vi "Begin.vi"(8 "error in":errorcluster) -> (0 "error out":errorcluster)   [LabVIEW 2015]
doc: "Called before other user functions, this VI is expected to open initial I/O refnums, load in file data, and do all program initialization. Notice that the <B>error out</B> terminal is simply used for data flow. Wiring it to other structures or subVIs ensures that this VI runs first."
uses:
  <vilib>/Rock Robotics/SystemInterfaces/DIO/FPGA_DIOPWMChannel.ctl
  <vilib>/Rock Robotics/WPI/SafetyOutput/WPI_SafetyOutputConfigMenu.ctl
  <vilib>/Rock Robotics/WPI/DriverStation/WPI_DriverStationRobotMode2.ctl
  <vilib>/Rock Robotics/WPI/Joystick/WPI_JoystickDeviceEnum.ctl
  <vilib>/Rock Robotics/SystemInterfaces/DIO/FPGA_DIOChannel.ctl
  <vilib>/Rock Robotics/WPI/Encoder/WPI_EncoderType.ctl
  <vilib>/Rock Robotics/WPI/RobotDrive/WPI_RobotDriveOpen2MotorWithTalon.vi
  Robot Global Data.vi
  <vilib>/Rock Robotics/Network Tables/NT Write String Array.vi
  <vilib>/Rock Robotics/WPI/Counter/WPI_CounterDigitalInputToDigitalSource.vi
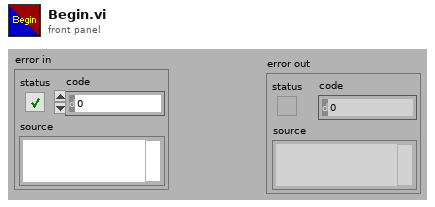
[diagram p1: front panel]
types:
  T1 = typedef "WPI_JoystickDeviceEnum.ctl" = enum16{"USB 0", "USB 1", "USB 2", "USB 3", "USB 4", "USB 5"}
  T2 = typedef "WPI_EncoderType.ctl" = enum16{"1x", "2x", "4x"}
  T3 = typedef "FPGA_DIOChannel.ctl" = enum8{"DIO 0", "DIO 1", "DIO 2", "DIO 3", "DIO 4", "DIO 5", "DIO 6", "DIO 7", "DIO 8", "DIO 9", "DIO MXP 0", "DIO MXP 1", "DIO MXP 2", "DIO MXP 3", "DIO MXP 4", "DIO MXP 5", "DIO MXP 6", "DIO MXP 7", "DIO MXP 8", "DIO MXP 9", "DIO MXP 10", "DIO MXP 11", "DIO MXP 12", "DIO MXP 13", "DIO MXP 14", "DIO MXP 15", "Invalid"}
  T4 = typedef "WPI_DriverStationRobotMode2.ctl" = enum16{"Autonomous Disabled", "Autonomous Enabled", "Teleop Disabled", "Teleop Enabled", "Disconnected", "Finish", "Test Disabled", "Test Enabled", "Emergency Stopped"}
  T5 = typedef "WPI_SafetyOutputConfigMenu.ctl" = enum16{"Enable", "Disable"}
  T6 = typedef "FPGA_DIOPWMChannel.ctl" = enum8{"PWM 0", "PWM 1", "PWM 2", "PWM 3", "PWM 4", "PWM 5", "PWM 6", "PWM 7", "PWM 8", "PWM 9", "PWM MXP 0", "PWM MXP 1", "PWM MXP 2", "PWM MXP 3", "PWM MXP 4", "PWM MXP 5", "PWM MXP 6", "PWM MXP 7", "PWM MXP 8", "PWM MXP 9", "Invalid"}
  T7 = typedef "WPI_JoystickDevRef.ctl" = cluster{"Device":T1}
  T8 = typedef "WPI_RobotDriveDevRef.ctl" = cluster{"DevStatus":errorcluster, "Motors[]":T9[], "Square Inputs":bool, "Max Output":dbl}
  T9 = typedef "WPI_MotorControlDeviceRef.ctl" = cluster{"DeviceStatus":errorcluster, "Type":T10, "PWM":cluster{"PWM Channel":T6, "DeadBand":T11}, "CAN":cluster{"Device Number":u8, "Control Mode":T12, "Semaphore":T13, "Max Vout":dbl, "TalonSRX Control Mode":T14}, "Invert":bool}
  T10 = typedef "WPI_MotorControlType.ctl" = enum16{"PWM", "CAN", "CANTalonSRX"}
  T11 = typedef "WPI_PWMDeadband.ctl" = cluster{"Name":string, "maxPositivePwm":i32, "minPositivePwm":i32, "centerPwm":i32, "maxNegativePwm":i32, "minNegativePwm":i32, "angularRange":u16}
  T12 = typedef "WPI_CANJaguar_ControlMode.ctl" = enum8{"Percent VBus", "Current", "Speed", "Position", "Voltage"}
  T13 = typedef "Semaphore RefNum" = refnum<k1>
  T14 = typedef "WPI_CANTalonSRX_APIControlMode.ctl" = enum8{"Percent VBus", "Speed", "Position", "Slave", "Unchanged / Invalid", "Voltage Compensation", "Current", "Motion Profile"}
  T15 = typedef "WPI_DigitalInputDevRef.ctl" = cluster{"DevStatus":errorcluster, "DIO Channel":T3}
  T16 = typedef "FPGA_CounterEncoderSourceConvertionLVSourceType.ctl" = cluster{"DevStatus":errorcluster, "AnalogTriggerMode?":bool, "DigitalMode":cluster{"DIO Channel":T17}, "AnalogTriggerMode":cluster{"AnalogTriggerIndex":T18, "OutputType":T19}}
  T17 = typedef "FPGA_DIODigitalSourceChannel.ctl" = enum8{"DIO 0", "DIO 1", "DIO 2", "DIO 3", "DIO 4", "DIO 5", "DIO 6", "DIO 7", "DIO 8", "DIO 9", "DIO MXP 0", "DIO MXP 1", "DIO MXP 2", "DIO MXP 3", "DIO MXP 4", "DIO MXP 5", "DIO MXP 6", "DIO MXP 7", "DIO MXP 8", "DIO MXP 9", "DIO MXP 10", "DIO MXP 11", "DIO MXP 12", "DIO MXP 13", "DIO MXP 14", "DIO MXP 15", "Disabled"}
  T18 = typedef "FPGA_AnalogTriggerIndex.ctl" = enum8{"Trig 0", "Trig 1", "Trig 2", "Trig 3", "Trig 4", "Trig 5", "Trig 6", "Trig 7", "Invalid"}
  T19 = typedef "FPGA_AnalogTriggerOutType.ctl" = enum16{"InWindow", "TriggerState", "Rising", "Falling"}
  T20 = typedef "WPI_EncoderDevRef.ctl" = cluster{"DevStatus":errorcluster, "EncoderIndex":T21, "CounterIndex":T22, "DistancePerCount":dbl, "Decoding Type":T2}
  T21 = typedef "FPGA_EncoderIdx.ctl" = enum8{"Enc 0", "Enc 1", "Enc 2", "Enc 3", "Enc 4", "Enc 5", "Enc 6", "Enc 7", "Invalid"}
  T22 = typedef "FPGA_CounterCtrSystemIndex.ctl" = enum8{"Ctr 0", "Ctr 1", "Ctr 2", "Ctr 3", "Ctr 4", "Ctr 5", "Ctr 6", "Ctr 7", "Invalid"}
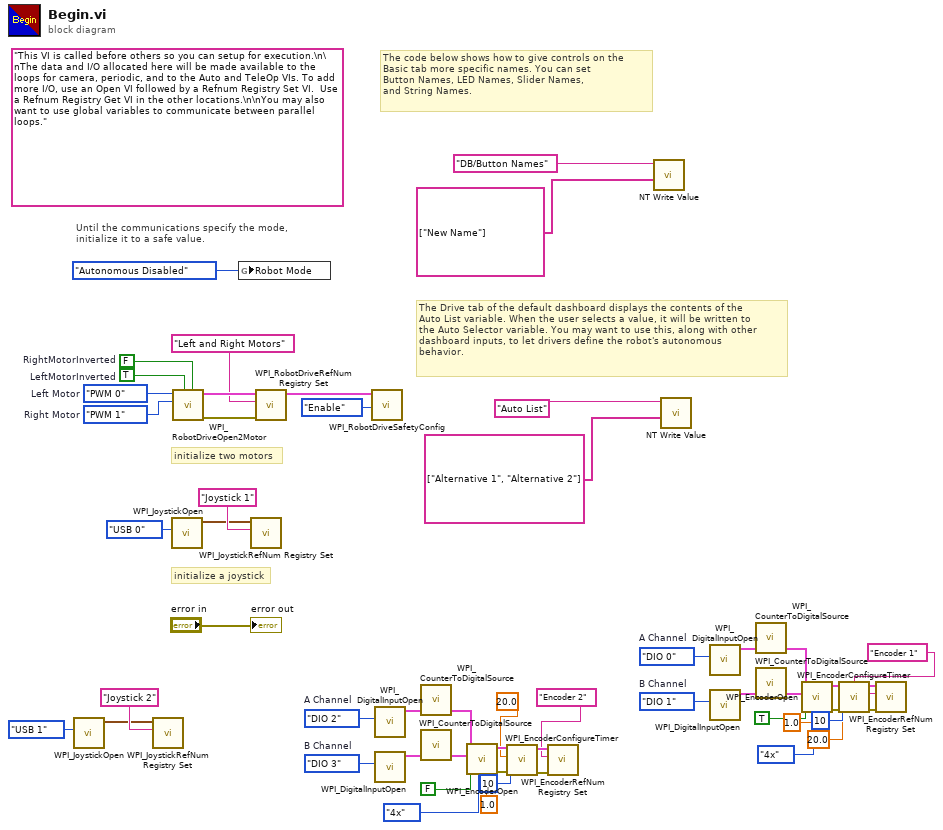
[diagram p0: block diagram]
diagram:
  w19 = FPGA_DIOChannel."DIO 3"  # B Channel
  w18 = FPGA_DIOChannel."DIO 2"  # A Channel
  w35 = FPGA_DIOChannel."DIO 1"  # B Channel
  w34 = FPGA_DIOChannel."DIO 0"  # A Channel
  (unwired) "This VI is called before others so you can setup for execution.\n\nThe data and I/O allocated here will be made available to the loops for camera, periodic, and to the Auto and TeleOp VIs. To add more I/O, use an Open VI followed by a Refnum Registry Set VI.  Use a Refnum Registry Get VI in the other locations.\n\nYou may also want to use global variables to communicate between parallel loops."
  w47 = FPGA_DIOPWMChannel."PWM 1"  # Right Motor
  w48 = FPGA_DIOPWMChannel."PWM 0"  # Left Motor
  w52 = TRUE  # LeftMotorInverted
  w53 = FALSE  # RightMotorInverted
  # "The Drive tab of the default dashboard displays the contents of the\nAuto List variable. When the user selects a value, it will be written to\nthe Auto Selector variable. You may want to use this, along with other\ndashboard inputs, to let drivers define the robot's autonomous\nbehavior."
  # "The code below shows how to give controls on the\nBasic tab more specific names. You can set\nButton Names, LED Names, Slider Names,\nand String Names."
  # "initialize a joystick"
  # "Until the communications specify the mode,\ninitialize it to a safe value."
  # "initialize two motors"
  n1 = call <vilib>:"WPI_JoystickOpen.vi"("JoystickDevice"=WPI_JoystickDeviceEnum."USB 1") -> ("JoystickDevRef"=w2:T7)  [unwired: 10 in]
  n2 = call <vilib>:"WPI_JoystickRefNum Registry Set.vi"("refnum name"="Joystick 2", "JoystickDevRef"=w2) -> ()  [unwired: 8 in, 2 out]
  n3 = call <vilib>:"WPI_JoystickOpen.vi"("JoystickDevice"=WPI_JoystickDeviceEnum."USB 0") -> ("JoystickDevRef"=w42:T7)  [unwired: 10 in]
  n4 = call-poly <vilib>:"WPI_RobotDriveOpen2Motor.vi"("Right Motor Inverted"=w53, "Left Motor Inverted"=w52, "Right Motor"=w47, "Left Motor"=w48) -> ("error out"=w49:errorcluster, "RobotDriveDevRef"=w51:T8)  [unwired: 1 in, 5 out]
  n5 = global write "Robot Global Data.vi" "Robot Mode"(WPI_DriverStationRobotMode2."Autonomous Disabled" ("Robot Mode")) -> ()
  n6 = call <vilib>:"WPI_JoystickRefNum Registry Set.vi"("refnum name"="Joystick 1", "JoystickDevRef"=w42) -> ()  [unwired: 8 in, 2 out]
  n7 = call <vilib>:"WPI_RobotDriveRefNum Registry Set.vi"("error in (no error)"=w49, "refnum name"="Left and Right Motors", "RobotDriveDevRef"=w51) -> ("RobotDriveDevRef"=w46:T8)  [unwired: 1 in, 7 out]
  n8 = call <vilib>:"WPI_RobotDriveSafetyConfig.vi"("mode"=WPI_SafetyOutputConfigMenu."Enable", "RobotDriveDevRef"=w46) -> ()  [unwired: 8 in, 2 out]
  n9 = call <vilib>:"WPI_DigitalInputOpen.vi"("DIO Channel"=w18) -> ("DigitalInputDevRef"=w15:T15)  [unwired: 1 in, 9 out]
  n10 = call <vilib>:"WPI_DigitalInputOpen.vi"("DIO Channel"=w19) -> ("DigitalInputDevRef"=w16:T15)  [unwired: 1 in, 9 out]
  n11 = call-poly <vilib>:"WPI_CounterToDigitalSource.vi"("DigitalInputDevRef"=w15) -> ("Digital Source"=w14:T16)  [unwired: 6 out]
  n12 = call-poly <vilib>:"WPI_CounterToDigitalSource.vi"("DigitalInputDevRef"=w16) -> ("Digital Source"=w17:T16)  [unwired: 6 out]
  n13 = call <vilib>:"WPI_EncoderOpen.vi"("DistancePerCount"=1.0, "Decoding Type"=WPI_EncoderType."4x", "Invert Direction (False)"=FALSE, "BSource"=w17, "ASource"=w14) -> ("error out"=w10:errorcluster, "EncoderDevRef"=w9:T20)  [unwired: 3 in, 2 out]
  n14 = call <vilib>:"WPI_EncoderConfigureTimer.vi"("error in (no error)"=w10, "Number Samples to Average"=u8 10, "Minimum Rate"=20.0, "EncoderDevRef"=w9) -> ("error out"=w6:errorcluster, "EncoderDevRef"=w5:T20)  [unwired: 6 in]
  n15 = call <vilib>:"WPI_EncoderRefNum Registry Set.vi"("error in (no error)"=w6, "refnum name"="Encoder 2", "EncoderDevRef"=w5) -> ()  [unwired: 7 in, 2 out]
  n16 = call-poly <vilib>:"NT Write Value.vi"("String Array"=string[] ["New Name"], "Name"="DB/Button Names") -> ()  [unwired: 9 in, 1 out]
  n17 = call-poly <vilib>:"NT Write Value.vi"("String Array"=string[] ["Alternative 1", "Alternative 2"], "Name"="Auto List") -> ()  [unwired: 9 in, 1 out]
  n18 = call <vilib>:"WPI_DigitalInputOpen.vi"("DIO Channel"=w34) -> ("DigitalInputDevRef"=w31:T15)  [unwired: 1 in, 9 out]
  n19 = call <vilib>:"WPI_DigitalInputOpen.vi"("DIO Channel"=w35) -> ("DigitalInputDevRef"=w32:T15)  [unwired: 1 in, 9 out]
  n20 = call-poly <vilib>:"WPI_CounterToDigitalSource.vi"("DigitalInputDevRef"=w31) -> ("Digital Source"=w30:T16)  [unwired: 6 out]
  n21 = call-poly <vilib>:"WPI_CounterToDigitalSource.vi"("DigitalInputDevRef"=w32) -> ("Digital Source"=w33:T16)  [unwired: 6 out]
  n22 = call <vilib>:"WPI_EncoderOpen.vi"("DistancePerCount"=1.0, "Decoding Type"=WPI_EncoderType."4x", "Invert Direction (False)"=TRUE, "BSource"=w33, "ASource"=w30) -> ("error out"=w26:errorcluster, "EncoderDevRef"=w25:T20)  [unwired: 3 in, 2 out]
  n23 = call <vilib>:"WPI_EncoderConfigureTimer.vi"("error in (no error)"=w26, "Number Samples to Average"=u8 10, "Minimum Rate"=20.0, "EncoderDevRef"=w25) -> ("error out"=w22:errorcluster, "EncoderDevRef"=w21:T20)  [unwired: 6 in]
  n24 = call <vilib>:"WPI_EncoderRefNum Registry Set.vi"("error in (no error)"=w22, "refnum name"="Encoder 1", "EncoderDevRef"=w21) -> ()  [unwired: 7 in, 2 out]
  "error out" <- "error in"
